vi "ep_Check Input Size.vi"(7 "check? (F)":bool, 8 "error in (no error)":errorcluster, 9 "array size of nameplate data":i32, 10 "algorithm":T1=enum."3-phase signals", 11 "number of channels":i32) -> (0 "error out":errorcluster, 3 "number of speed":i32)   [LabVIEW 2014, in "NI_EP_Motor Monitoring.lvlib"]
uses:
  <vilib>/addons/Electrical Power/Motor Monitoring/NI_EP_Motor Monitoring.lvlib
  <vilib>/addons/Electrical Power/Motor Monitoring/subVIs/ep_Demodulation Algorithm.ctl
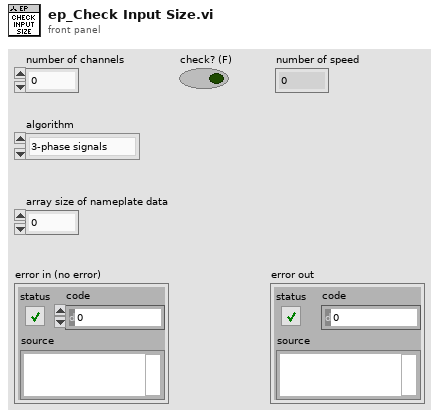
[diagram p1: front panel]
types:
  T1 = typedef "NI_EP_Motor Monitoring.lvlib/ep_Demodulation Algorithm.ctl" = enum16{"1-phase signal", "3-phase signals"}
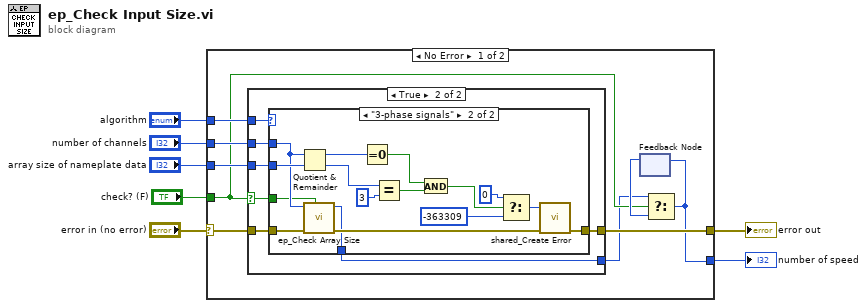
[diagram p0: block diagram]
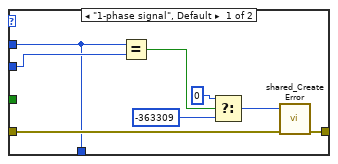
[diagram p3: hidden frame]
diagram:
  n1 = case shown="No Error" "error in (no error)" {
    selector: "error in (no error)" -> [w12 w49]
    tunnel: "number of channels" -> [w13 _]
    tunnel: "algorithm" -> [w14 _]
    tunnel: [w15 w49] -> w4
    tunnel: "array size of nameplate data" -> [w16 _]
    tunnel: [w8 _] -> w2
    tunnel: "check? (F)" -> [w10 _]
    frame No Error {
      n2 = case shown="True" w10 {
        selector: w10 -> [_ w18]
        tunnel: w16 -> [_ w24]
        tunnel: [w17 w23] -> w15
        tunnel: w14 -> [_ w22]
        tunnel: w13 -> [_ w21]
        tunnel: [_ w20] -> w9
        tunnel: w12 -> [w17 w19]
        frame False {
        }
        frame True {
          n3 = case shown="\"3-phase signals\"" w22 {
            tunnel: w21 -> [w25 w35]
            tunnel: w19 -> [w28 w37]
            tunnel: w24 -> [w26 w39]
            tunnel: [w27 w38] -> w23
            tunnel: [w25 w34] -> w20
            tunnel: w18 -> [_ w33]
            frame "1-phase signal", Default {
              n4 = Equal?(x=w25, y=w26) -> (x = y?=w29:bool)
              n5 = Select(t=0 ("y"), s=w29, f=-363309 ("y")) -> (s? t:f=w30:i32)
              n6 = call <vilib>:"shared_Create Error.vi"("error in (no error)"=w28, "error code (0)"=w30) -> ("error out"=w27:errorcluster)  [unwired: 9 in]
            }
            frame "3-phase signals" {
              n7 = Quotient & Remainder(x=w35, y=w39) -> (x-y*floor(x/y)=w48:i32, floor(x/y)=w47:i32)
              n8 = call <vilib>:"ep_Check Array Size.vi"("reset? (F)"=w33, "error in (no error)"=w37, "number of channels"=w35) -> ("error out"=w36:errorcluster, "number of spectra"=w34:i32)  [unwired: 7 in]
              n9 = Equal To 0?(x=w48) -> (x = 0?=w45:bool)
              n10 = Equal?(x=w47, y=3) -> (x = y?=w44:bool)
              n11 = And(x=w45, y=w44) -> (x .and. y?=w43:bool)
              n12 = Select(t=0 ("y"), s=w43, f=-363309 ("y")) -> (s? t:f=w40:i32)
              n13 = call <vilib>:"shared_Create Error.vi"("error in (no error)"=w36, "error code (0)"=w40) -> ("error out"=w38:errorcluster)  [unwired: 9 in]
            }
          }
        }
      }
      n14 = feedback #1() -> (w11:i32)  [unwired: 1 in]
      n15 = Select(t=w9, s=w10, f=w11) -> (s? t:f=w8:i32)
      n16 = feedback-in #1(w8) -> ()
    }
    frame Error {
    }
  }
  "error out" <- w4
  "number of speed" <- w2
